vi "Read Mode.vi"(8 "error in (no error)":errorcluster, 11 "MB_Serial_Master in":refnum<class "MB_Master_Serial.lvclass">) -> (0 "error out":errorcluster, 2 "Mode":enum16{"RTU", "ASCII"}(ring), 3 "MB_Serial_Master out":refnum<class "MB_Master_Serial.lvclass">)   [LabVIEW 2016, in "MB Master.lvlib" / "MB_Master_Serial.lvclass"]
uses:
  MB_Master_Serial.lvclass
  MB_Master_Serial.lvclass/MB_Master_Serial.ctl
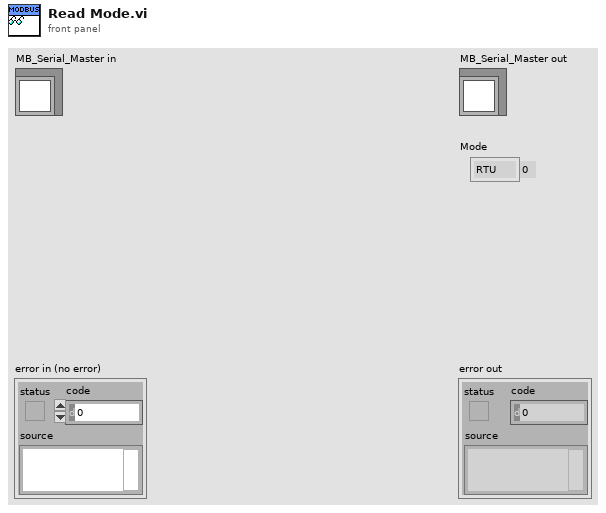
[diagram p1: front panel]
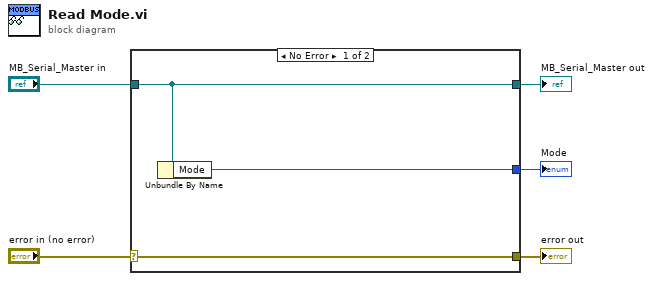
[diagram p0: block diagram]
diagram:
  n1 = case shown="No Error" "error in (no error)" {
    selector: "error in (no error)" -> [w8 w9]
    tunnel: [w8 w9] -> w4
    tunnel: [w7 w10] -> w2
    tunnel: "MB_Serial_Master in" -> [w7 w10]
    tunnel: [w6 _] -> w1
    frame No Error {
      n2 = Unbundle By Name(w7) -> ("Mode"=w6:enum16{"RTU", "ASCII"})
    }
    frame Error {
    }
  }
  "error out" <- w4
  "MB_Serial_Master out" <- w2
  "Mode" <- w1
